vi "listbox_set_translated_values.vi"(4 "item_names":string[][](array[string]), 6 "front_panel_reference":refnum<vi>, 7 "column_names":string[](array[string]), 8 "error_in":errorcluster, 9 "Autosize? (T)":bool=TRUE, 11 "multicolumn_listbox_reference_in":refnum<vi>) -> (0 "error_out":errorcluster, 3 "multicolumn_listbox_reference_out":refnum<vi>)   [LabVIEW 2019]
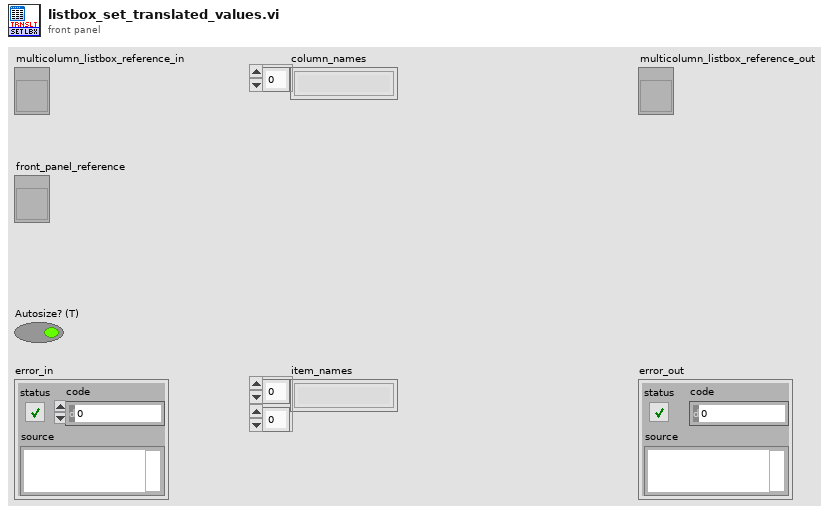
[diagram p1: front panel]
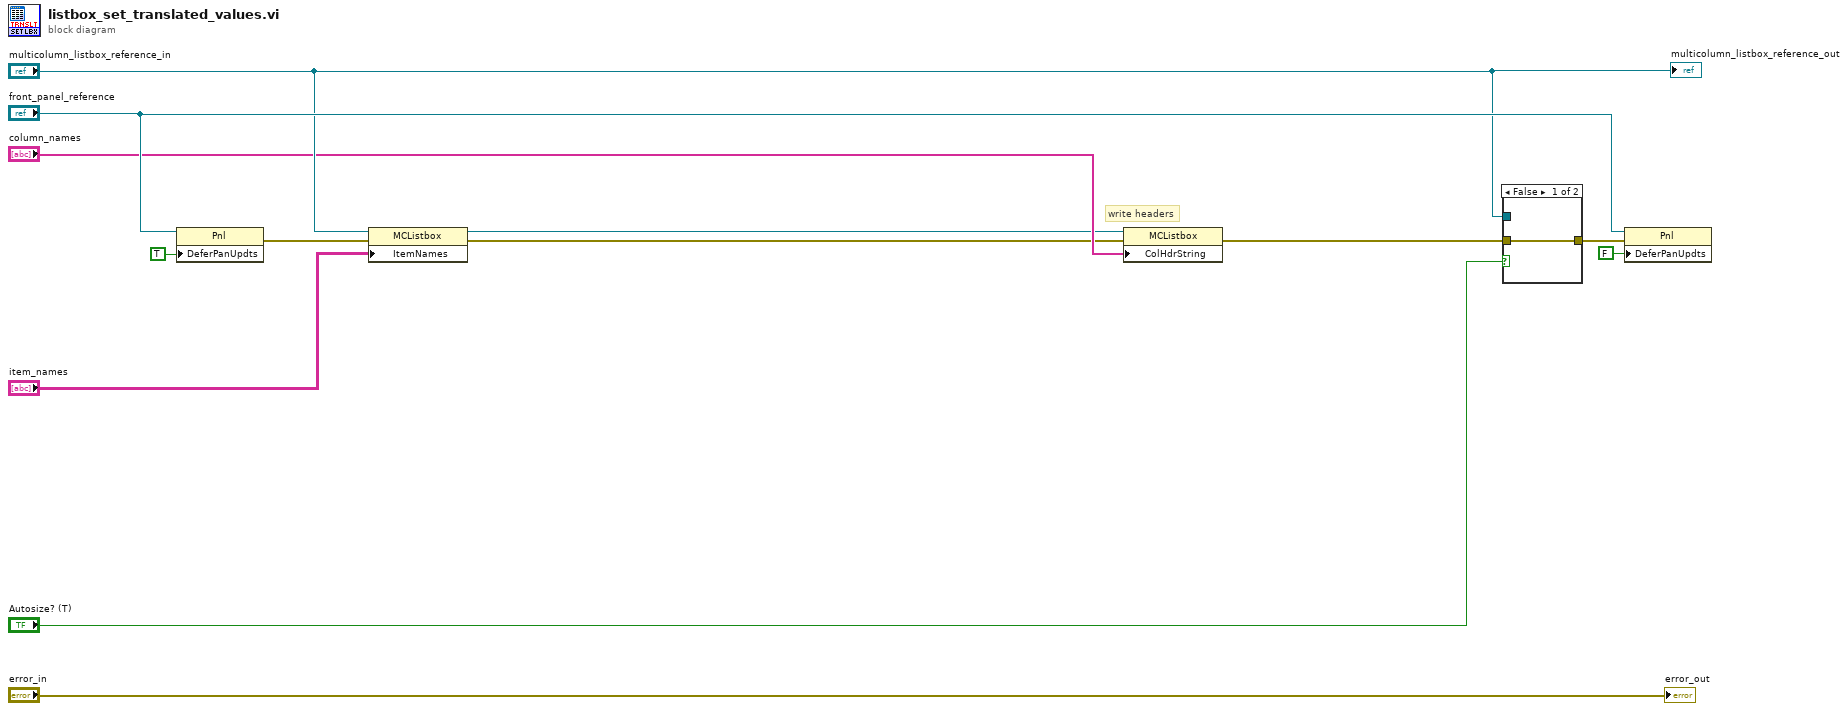
[diagram p0: block diagram]
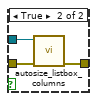
[diagram p2: hidden frame]
diagram:
  # "write headers"
  n1 = property on="Property Node" class="Pnl"(reference="front_panel_reference", "DeferPanUpdts"=TRUE ("Defer Panel Updates")) -> (error out=w9:errorcluster)  [unwired: 1 in, 1 out]
  n2 = property on="Property Node" class="MCListbox"(reference="multicolumn_listbox_reference_in", error in=w9, "ItemNames"="item_names") -> (reference out=w5:refnum<vi>, error out=w2:errorcluster)
  n3 = property on="Property Node" class="MCListbox"(reference=w5, error in=w2, "ColHdrString"="column_names") -> (error out=w1:errorcluster)  [unwired: 1 out]
  n4 = case shown="False" "Autosize? (T)" {
    tunnel: w1 -> [w14 w17]
    tunnel: [w14 w16] -> w8
    tunnel: "multicolumn_listbox_reference_in" -> [_ w15]
    frame False {
    }
    frame True {
      n5 = call "autosize_listbox_columns.vi"("error in (no error)"=w17, "Table Ref"=w15) -> ("error out"=w16:errorcluster)  [unwired: 4 in, 1 out]
    }
  }
  n6 = property on="Property Node" class="Pnl"(reference="front_panel_reference", error in=w8, "DeferPanUpdts"=FALSE ("Defer Panel Updates")) -> ()  [unwired: 2 out]
  "error_out" <- "error_in"
  "multicolumn_listbox_reference_out" <- "multicolumn_listbox_reference_in"
